vi "Process.vi"(0 "Process In":refnum<class "Message Handler.lvclass">, 11 "Error In":errorcluster) -> (4 "Process Out":refnum<class "Message Handler.lvclass">, 15 "Error Out":errorcluster)   [LabVIEW 2023, in "Message Handler.lvclass"]
uses:
  Message Handler.lvclass
  Private/Ctrls/Process Variables.ctl
  Interfaces/ICanCommunicate/ICanCommunicate.lvclass
  Interfaces/ICanCommunicate/Process Refs.ctl
  Interfaces/ICanCommunicate/ToProcessQueue.ctl
  Interfaces/ICanCommunicate/Message.ctl
  Interfaces/ICanCommunicate/FromProcessQueue.ctl
  Interfaces/ICanCommunicate/ProcessSyncQueue.ctl
  Private/Ctrls/Registration Data.ctl
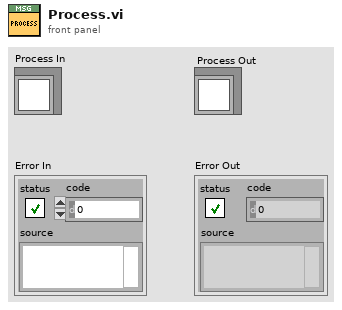
[diagram p1: front panel]
types:
  T1 = typedef "ICanCommunicate.lvclass/Message.ctl" = cluster{"Sender Name":string, "Recipent Name":string, "Command":string, "Data":variant, "Signature":string}
  T2 = typedef "Message Handler.lvclass/Process Variables.ctl" = cluster{"Recipents":map{refnum<class "ICanCommunicate.lvclass">, T3}}
  T3 = typedef "ICanCommunicate.lvclass/Process Refs.ctl" = cluster{"ToProcessQueue":T4, "FromProcessQueue":T5, "ProcessSyncQueue":T6, "ProcessViRef":refnum<vi>}
  T4 = typedef "ICanCommunicate.lvclass/ToProcessQueue.ctl" = refnum<queue>
  T5 = typedef "ICanCommunicate.lvclass/FromProcessQueue.ctl" = refnum<queue>
  T6 = typedef "ICanCommunicate.lvclass/ProcessSyncQueue.ctl" = refnum<queue>
  T7 = typedef "Message Handler.lvclass/Registration Data.ctl" = cluster{"ICanCommunicate":refnum<class "ICanCommunicate.lvclass">, "ProcessRefs":T3}
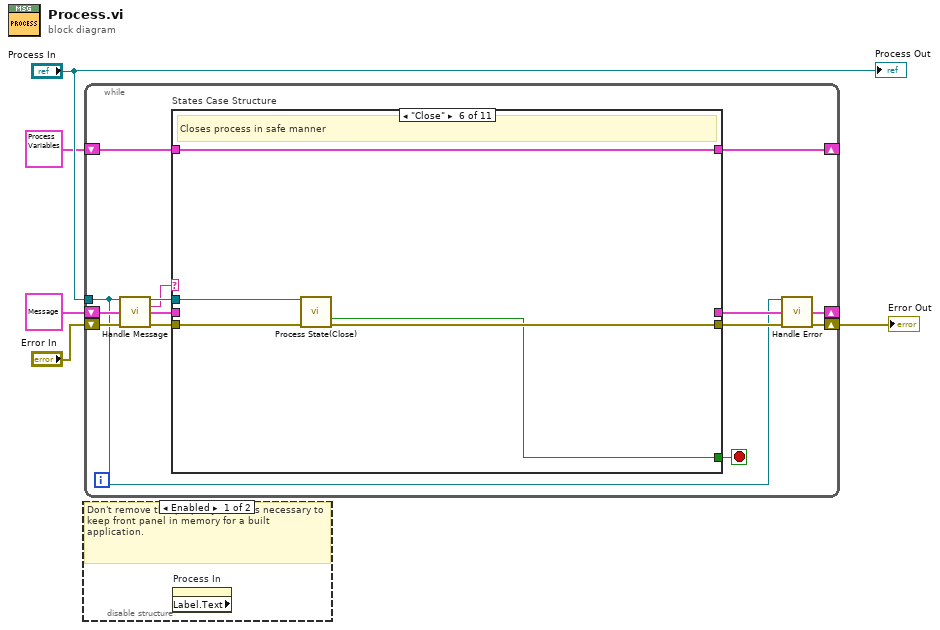
[diagram p0: block diagram]
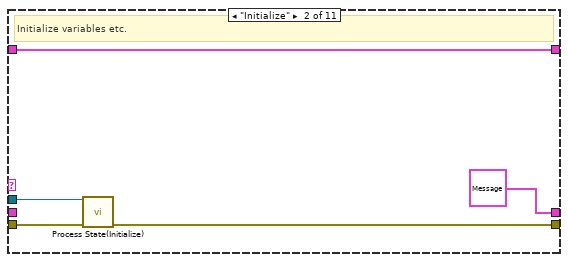
[diagram p4: hidden frame]
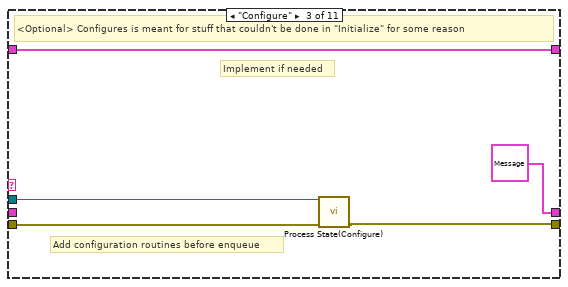
[diagram p5: hidden frame]
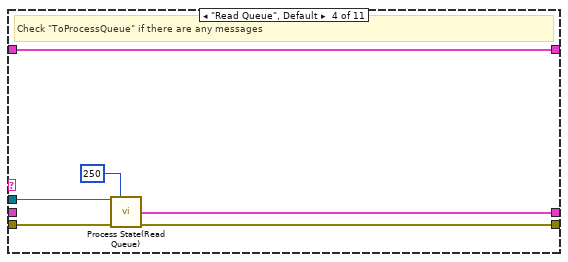
[diagram p6: hidden frame]
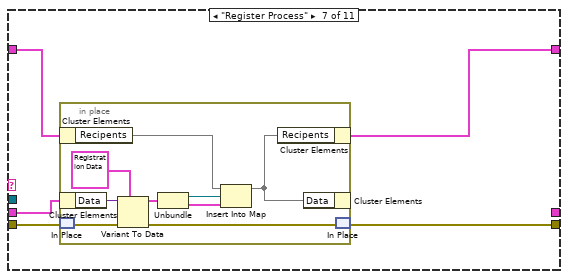
[diagram p8: hidden frame]
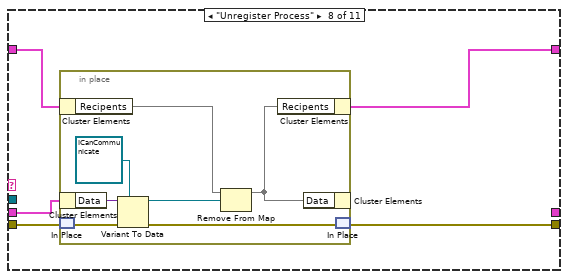
[diagram p9: hidden frame]
diagram:
  n1 = disable-structure shown="Enabled" {
    frame Enabled {
      # "Don't remove this property node it's necessary to keep front panel in memory for a built application."
      n2 = property on="Process In" class="LVClassControl (strict)" props=["Label", "Text"]() -> ()  [unwired: 2 in, 3 out]
    }
    frame Disabled {
    }
  }
  n3 = while {
    shift-right: [w9] -> w5
    shift-left: "Error In" -> [w15]
    tunnel: "Process In" -> [w6]
    shift-right: [w18] -> _
    shift-left: T2 {"Recipents"={}} ("Process Variables") -> [w17]
    shift-right: [w7] -> _
    shift-left: T1 {"Sender Name"="", "Recipent Name"="", "Command"="Initialize", "Data"=variant, "Signature"=""} ("Message") -> [w12]
    stop <- w16 stop-if-true
    n4 = call-dynamic "Handle Message.vi"("Message Handler In"=w6, "Message In"=w12, "Error In"=w15) -> ("Message Handler Out"=w11:refnum<class "Message Handler.lvclass">, "CMD Out"=w10:string, "Message Out"=w13:T1, "Error Out"=w14:errorcluster)  [unwired: 9 in]
    n5 = case "States Case Structure" shown="\"Close\"" w10 {
      tunnel: w14 -> [w22 w25 w30 w37 w41 w45 w49 w63 w75 w78 w81]
      tunnel: [w22 w23 w28 w36 w41 w43 w48 w62 w75 w78 w81] -> w19
      tunnel: [w21 w27 w32 w38 w40 w46 w47 w61 w74 w77 w80] -> w18
      tunnel: w17 -> [w21 w27 w32 w38 w40 w46 w51 w65 w74 w77 w80]
      tunnel: [_ _ _ _ _ w42 _ _ _ _ _] -> w16
      tunnel: w13 -> [w20 _ _ _ w39 _ w50 w64 w73 w76 w79]
      tunnel: [w20 T1 {"Sender Name"="", "Recipent Name"="", "Command"="Start Message Handler", "Data"=variant, "Signature"=""} ("Message") T1 {"Sender Name"="", "Recipent Name"="", "Command"="Read Queue", "Data"=variant, "Signature"=""} ("Message") w35 w39 _ _ _ w73 w76 w79] -> w8
      tunnel: w11 -> [_ w24 w29 w34 _ w44 _ _ _ _ _]
      frame "--- Common ---" {
        # "Only for grouping"
      }
      frame "Initialize" {
        # "Initialize variables etc."
        n6 = call-dynamic "Process State(Initialize).vi"("Process In"=w24, "Error In"=w25) -> ("Error Out"=w23:errorcluster)  [unwired: 12 in, 1 out]
      }
      frame "Configure" {
        # "Implement if needed"
        # "Add configuration routines before enqueue"
        # "<Optional> Configures is meant for stuff that couldn't be done in \"Initialize\" for some reason"
        n7 = call-dynamic "Process State(Configure).vi"("Process In"=w29, "Error In"=w30) -> ("Error Out"=w28:errorcluster)  [unwired: 12 in, 1 out]
      }
      frame "Read Queue", Default {
        # "Check \"ToProcessQueue\" if there are any messages"
        n8 = call-dynamic "Process State(Read Queue).vi"("Process In"=w34, "Timeout in ms (-1)"=250, "Error In"=w37) -> ("Message"=w35:T1, "Error Out"=w36:errorcluster)  [unwired: 9 in, 2 out]
      }
      frame "Timeout" {
        # "<Optional> Actions to be taken if there are no messages for process"
      }
      frame "Close" {
        # "Closes process in safe manner"
        n9 = call-dynamic "Process State(Close).vi"("Process In"=w44, "Error In"=w45) -> ("Close?"=w42:bool, "Error Out"=w43:errorcluster)  [unwired: 11 in, 1 out]
      }
      frame "Register Process" {
        n10 = in-place {
          n11 = in-place-cluster #1(w51) -> ("Recipents"=w57:map{refnum<class "ICanCommunicate.lvclass">, T3})
          n12 = in-place-cluster #2(w50) -> ("Data"=w60:variant)
          n13 = in-place-match #3(w49) -> (w54:errorcluster)
          n14 = Variant To Data(error in=w54, type=T7 {"ICanCommunicate"=refnum, "ProcessRefs"={"ToProcessQueue"=refnum, "FromProcessQueue"=refnum, "ProcessSyncQueue"=refnum, "ProcessViRef"=refnum}} ("Registration Data"), Variant=w60) -> (data=w58:T7, error out=w53:errorcluster)
          n15 = Unbundle(w58) -> ("ICanCommunicate"=w56:refnum<class "ICanCommunicate.lvclass">, "ProcessRefs"=w55:T3)
          n16 = Insert Into Map(map in=w57, key=w56, value=w55) -> (map out=w52:map{refnum<class "ICanCommunicate.lvclass">, T3})  [unwired: 2 out]
          n17 = in-place-cluster #1("Recipents"=w52) -> (w47:T2)
          n18 = in-place-cluster #2("Data"=w52) -> ()  [unwired: 1 out]
          n19 = in-place-match #3(w53) -> (w48:errorcluster)
        }
      }
      frame "Unregister Process" {
        n20 = in-place {
          n21 = in-place-cluster #4(w65) -> ("Recipents"=w68:map{refnum<class "ICanCommunicate.lvclass">, T3})
          n22 = in-place-cluster #5(w64) -> ("Data"=w72:variant)
          n23 = in-place-match #6(w63) -> (w71:errorcluster)
          n24 = Variant To Data(error in=w71, type=refnum<class "ICanCommunicate.lvclass"> refnum ("ICanCommunicate"), Variant=w72) -> (data=w67:refnum<class "ICanCommunicate.lvclass">, error out=w70:errorcluster)
          n25 = Remove From Map(10:w67, 11:w68) -> (3:w69:map{refnum<class "ICanCommunicate.lvclass">, T3})  [unwired: 2 out]
          n26 = in-place-cluster #4("Recipents"=w69) -> (w61:T2)
          n27 = in-place-cluster #5("Data"=w69) -> ()  [unwired: 1 out]
          n28 = in-place-match #6(w70) -> (w62:errorcluster)
        }
      }
      frame "Async. Message" {
      }
      frame "Async. Data Request" {
      }
      frame "Sync. Data Request" {
      }
    }
    n29 = call-dynamic "Handle Error.vi"("Process In"=w6, "Message In"=w8, "Error In"=w19) -> ("Message Out"=w7:T1, "Error Out"=w9:errorcluster)  [unwired: 10 in, 1 out]
  }
  "Error Out" <- w5
  "Process Out" <- "Process In"
